vi "ResonanceAnalyzer.vi"() -> ()   [LabVIEW 2014]
uses:
  <vilib>/imath/engines/lvmath/Plug In/_Char/NIMS_CH_character datatype.ctl
  <vilib>/imath/engines/lvmath2/RunTimeEngine/Managers/WorkSpace/UID Generator.vi
  <vilib>/imath/engines/lvmath2/RunTimeEngine/RunTimeType/NIMS_RunTimeType_From StrictType (excl LVString).vi
  <instcachedir>/0/NIMS_RunTimeType_From StrictType (excl LVString)_15A5391EEA9C4AACB9955AC755B83D29.lvgen/NIMS_RunTimeType_From StrictType (excl LVString)_15A5391EEA9C4AACB9955AC755B83D29_000.vi
  <vilib>/imath/engines/lvmath2/RunTimeEngine/LocalVariableDefStatement/MC_LocalVariableDefStatement_Display.vi
  <vilib>/imath/engines/lvmath2/RunTimeEngine/BuiltInFunctions/int32/NIMS_int32(real).vi
  <instcachedir>/0/NIMS_int32(real)_9F6AE75EF4BE45429513317A1C5A7040.lvgen/NIMS_int32(real)_9F6AE75EF4BE45429513317A1C5A7040_000.vi
  <vilib>/imath/engines/lvmath2/RunTimeEngine/BuiltInFunctions/linramp/NIMS_linramp.vi
  <vilib>/imath/engines/lvmath2/RunTimeEngine/RangeToken/NIMS_Range_R2 - Integer.vi
  <instcachedir>/0/NIMS_Range_R2 - Integer_2D1304BAF97744E0A293025746CBADFC.lvgen/NIMS_Range_R2 - Integer_2D1304BAF97744E0A293025746CBADFC_000.vi
  <vilib>/imath/engines/lvmath2/RunTimeEngine/CommandStatement/MC_CommandStatement_break.vi
  <vilib>/imath/engines/lvmath2/RunTimeEngine/IndexRead/NIMS V(S).vi
  <instcachedir>/0/NIMS V(S)_0488751826AF41519A22953C041130DC.lvgen/NIMS V(S)_0488751826AF41519A22953C041130DC_000.vi
  <vilib>/imath/engines/lvmath2/RunTimeEngine/IndexReplace/NIMS V(S)=S.vi
  <instcachedir>/0/NIMS V(S)=S_2D52C4EC15D8415E870AEE69FB516CCA.lvgen/NIMS V(S)=S_2D52C4EC15D8415E870AEE69FB516CCA_001.vi
  <vilib>/imath/engines/lvmath2/RunTimeEngine/ErrorHandling/NIMS_Create Error From Enums.vi
  <vilib>/imath/engines/lvmath/Plug In/_Char/NIMS_CH_Character RV to String.vi
  <instcachedir>/0/NIMS V(S)_0488751826AF41519A22953C041130DC.lvgen/NIMS V(S)_0488751826AF41519A22953C041130DC_003.vi
  <vilib>/imath/engines/lvmath2/RunTimeEngine/BuiltInFunctions/random/NIMS_random.vi
  <vilib>/imath/engines/lvmath2/RunTimeEngine/IndexReplace/NIMS V(S)=M.vi
  <instcachedir>/0/NIMS V(S)=M_608EF2A6197B4B6A9CB600D58D177061.lvgen/NIMS V(S)=M_608EF2A6197B4B6A9CB600D58D177061_001.vi
  <vilib>/imathl/engines/lvmath/Functions/Error Handling/Create Error.vi
  <vilib>/imath/engines/lvmath2/RunTimeEngine/BuiltInFunctions/and/NIMS_and.vi
  <instcachedir>/0/NIMS_and_04EBB299D59649339AD86944E4B9B28A.lvgen/NIMS_and_04EBB299D59649339AD86944E4B9B28A_000.vi
  <vilib>/imath/engines/lvmath/Functions/Error Handling/MergeErrorsWrapper.vi
  <vilib>/imath/engines/lvmath2/RunTimeEngine/Managers/SymbolTable/Clear UID.vi
  <vilib>/imath/engines/lvmath2/RunTimeEngine/NodeEndStatement/NIMS_NodeEndStatement_Output.vi
  <instcachedir>/0/NIMS_NodeEndStatement_Output_53EC0D466D134D7ABD903AC30B43404B.lvgen/NIMS_NodeEndStatement_Output_53EC0D466D134D7ABD903AC30B43404B_011.vi
  <instcachedir>/0/NIMS_NodeEndStatement_Output_53EC0D466D134D7ABD903AC30B43404B.lvgen/NIMS_NodeEndStatement_Output_53EC0D466D134D7ABD903AC30B43404B_001.vi
  <instcachedir>/0/NIMS_NodeEndStatement_Output_53EC0D466D134D7ABD903AC30B43404B.lvgen/NIMS_NodeEndStatement_Output_53EC0D466D134D7ABD903AC30B43404B_010.vi
  <instcachedir>/0/NIMS_NodeEndStatement_Output_53EC0D466D134D7ABD903AC30B43404B.lvgen/NIMS_NodeEndStatement_Output_53EC0D466D134D7ABD903AC30B43404B_000.vi
  <instcachedir>/0/NIMS_NodeEndStatement_Output_53EC0D466D134D7ABD903AC30B43404B.lvgen/NIMS_NodeEndStatement_Output_53EC0D466D134D7ABD903AC30B43404B_005.vi
  <vilib>/imath/engines/lvmath2/RunTimeEngine/ErrorHandling/NIMS_Finalize Error.vi
  <vilib>/imath/engines/lvmath2/RunTimeEngine/Managers/SymbolTable/NIMS_WorkSpace.lvlib
panel:
  out "rightindex":i32
  out "leftindex":i32
  out "Amp":cdb[](array[numeric])
  out "delta_f":dbl
  out "Results":T1
  in  "String":string="This is a text.\nHere is a new line.\n\nAnd that's another."
  out "XY Graph":cluster{"Freq":dbl[], "Amp":dbl[]}(graph)
  in  "Tab Control":enum32{"Simulation", "Experiment"}(tab)
  in  "Center Frequency":dbl=600.0
  in  "Q":dbl=10.0
  in  "Start Frequency":dbl=400.0
  in  "End Frequency":dbl=800.0
  in  "df":dbl=5.0
  in  "Noise Level":dbl=0.01
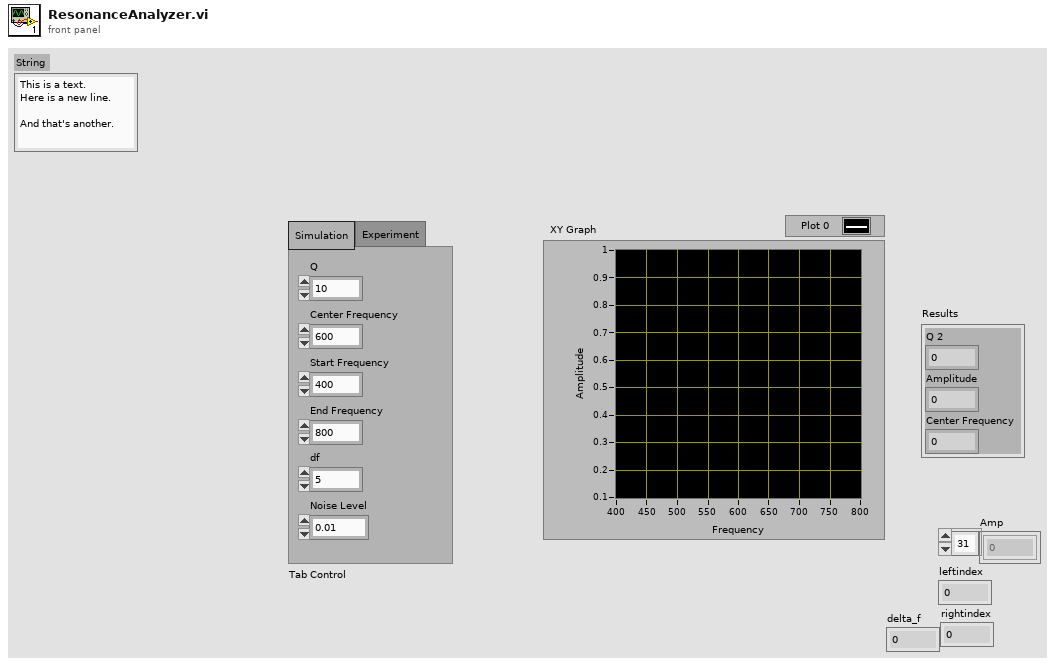
[diagram p1: front panel]
types:
  T1 = cluster{"Q 2":dbl, "Amplitude":dbl, "Center Frequency":dbl}
  T2 = typedef "NIMS_CH_character datatype.ctl" = cluster{"Numeric":u8}
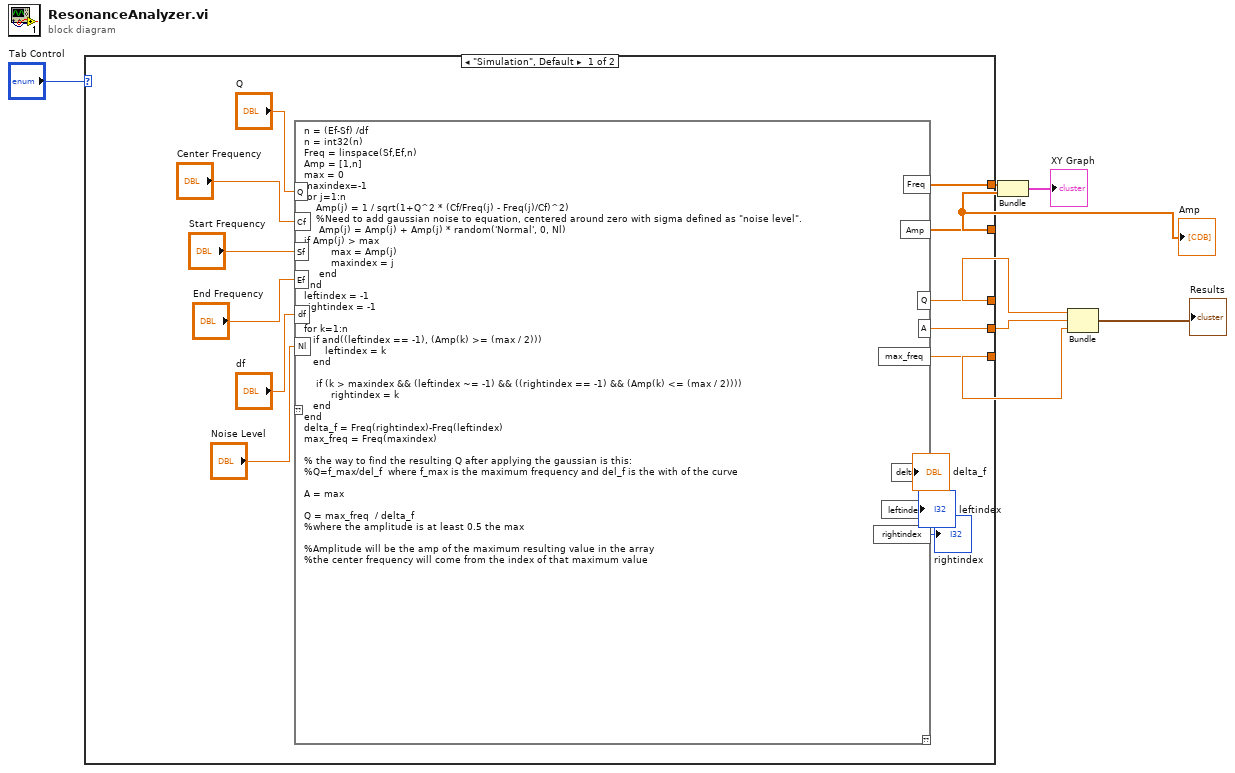
[diagram p0: block diagram]
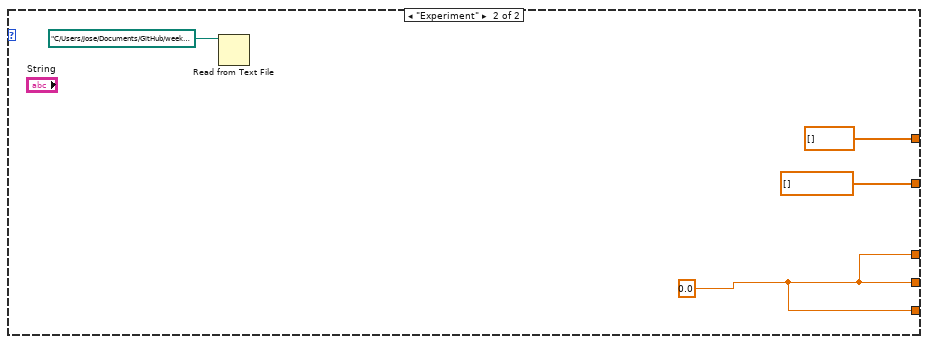
[diagram p2: hidden frame]
diagram:
  n1 = case shown="\"Simulation\", Default" "Tab Control" {
    tunnel: [w16 dbl[] [] ("Freq")] -> w7
    tunnel: [w15 cdb[] [] ("Amp")] -> w1
    tunnel: [w14 w678] -> w5
    tunnel: [w13 w678] -> w4
    tunnel: [w12 w678] -> w3
    frame "Simulation", Default {
      n2 = mathscript code="n = (Ef-Sf) /df\nn = int32(n)\nFreq = linspace(Sf,Ef,n)\nAmp = [1,n]\nmax = 0\nmaxindex=-1\nfor j=1:n\n    Amp(j) = 1 / sqrt(1+Q^2 * (Cf/Freq(j) - Freq(j)/Cf)^2)\n    %Need to add gaussian noise to equation, centered around zero with sigma defined as \"noise level\".\n     Amp(j) = Amp(j) + Amp(j) * random('Normal', 0, Nl)\nif Amp(j) > max\n         max = Amp(j)\n         maxindex = j\n     end\nend\nleftindex = -1\nrightindex = -1\n\nfor k=1:n\n   if and((leftindex == -1), (Amp(k) >= (max / 2)))\n       leftindex = k\n   end\n\n    if (k > maxindex && (leftindex ~= -1) && ((rightindex == -1) && (Amp(k) <= (max / 2))))\n         rightindex = k\n   end\nend\ndelta_f = Freq(rightindex)-Freq(leftindex)\nmax_freq = Freq(maxindex)\n\n% the way to find the resulting Q after applying the gaussian is this:\n%Q=f_max/del_f  where f_max is the maximum frequency and del_f is the with of the curve \n\nA = max\n\nQ = max_freq  / delta_f\n%where the amplitude is at least 0.5 the max\n\n%Amplitude will be the amp of the maximum resulting value in the array\n%the center frequency will come from the index of that maximum value"("Q"="Q", "Cf"="Center Frequency", "Sf"="Start Frequency", "Ef"="End Frequency", "df"="df", "Nl"="Noise Level") -> ("Freq"=w16:dbl[], "Amp"=w15:cdb[], "Q"=w14:dbl, "A"=w13:cdb, "max_freq"=w12:dbl, "delta_f"=→"delta_f":dbl, "leftindex"=→"leftindex":i32, "rightindex"=→"rightindex":i32)  [unwired: 1 in, 1 out]
    }
    frame "Experiment" {
      w678 = 0.0
      n3 = Read from Text File(file (use dialog)=path "C:/Users/Jose/Documents/GitHub/week5/output2.txt") -> ()  [unwired: 3 in, 4 out]
    }
  }
  "Amp" <- w1
  n4 = Bundle("Freq"=w7, "Amp"=w1) -> (→"XY Graph":cluster{"Freq":dbl[], "Amp":cdb[]})  [unwired: 1 in]
  n5 = Bundle("Q"=w5, "A"=w4, "max_freq"=w3) -> (→"Results":cluster{"Q":dbl, "A":cdb, "max_freq":dbl})  [unwired: 1 in]
